vi "Menu Actions.vi"(0 "queue in":refnum<queue>, 1 "LBCB Number":T1, 2 "menu reference":refnum<k9>, 3 "error in":errorcluster, 4 "ItemTag":string) -> (5 "queue out":refnum<queue>, 6 "error out":errorcluster)   [LabVIEW 2009]
uses:
  Data Access Objects/Metadata/LBCB Number.ctl
  Control Loop/Parameters Changes.ctl
  Control Loop/Parameter Change States.ctl
  App Status Actions.ctl
  Launcher/Launcher Actions.ctl
  Launcher/NoPanelAppTypes.ctl
  Data Access Objects/Metadata/Persistant DAO Actions.ctl
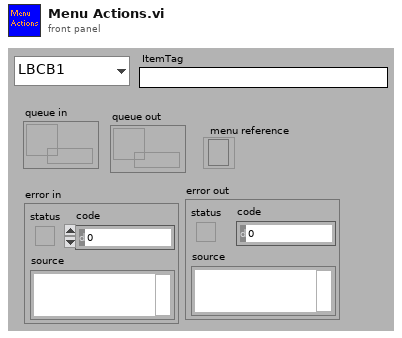
[diagram p1: front panel]
types:
  T1 = typedef "LBCB Number.ctl" = enum16{"LBCB1", "LBCB2"}
  T2 = typedef "Parameters Changes.ctl" = cluster{"Change State":T3, "LBCB Number":T1}
  T3 = typedef "Parameter Change States.ctl" = enum16{"Mixed Mode", "Control Loop", "Limits", "Application", "Stiffness Jacobian", "Start DAQ", "Auto-Balancing", "Set Command", "Enable Control", "Disable Control", "Stop Application"}
  T4 = typedef "App Status Actions.ctl" = enum16{"Init", "Get Status", "Running", "Control", "Autobalanced", "Data Acquisition", "Set App State", "DAQ Started", "Set LBCB State", "Set All", "Set Cont Logging", "Set Step Logging", "Set MM Logging", "Set Volt Logging", "Set Cart Type", "Set DAQ Link", "Set NTCP Link"}
  T5 = typedef "Launcher Actions.ctl" = enum16{"Launch", "Stop All", "Stop", "Kill", "Running?", "Init"}
  T6 = typedef "NoPanelAppTypes.ctl" = enum16{"NTCP Socket", "Data Archiving", "DAQ Link", "Control Loops", "Autobalance Monitor", "Mixed Mode Monitor", "Cmd Disp Diffs"}
  T7 = typedef "Persistant DAO Actions.ctl" = enum16{"Init", "Get", "Set", "Load", "Save"}
  T8 = typedef "LBCB Location.ctl" = enum16{"Crane Bay Two LBCB", "Crane Bay One LBCB", "5th Scale Two LBCB", "5th Scale One LBCB", "Portable LBCB"}
  T9 = typedef "Stiffness Matrix.ctl" = dbl[][]
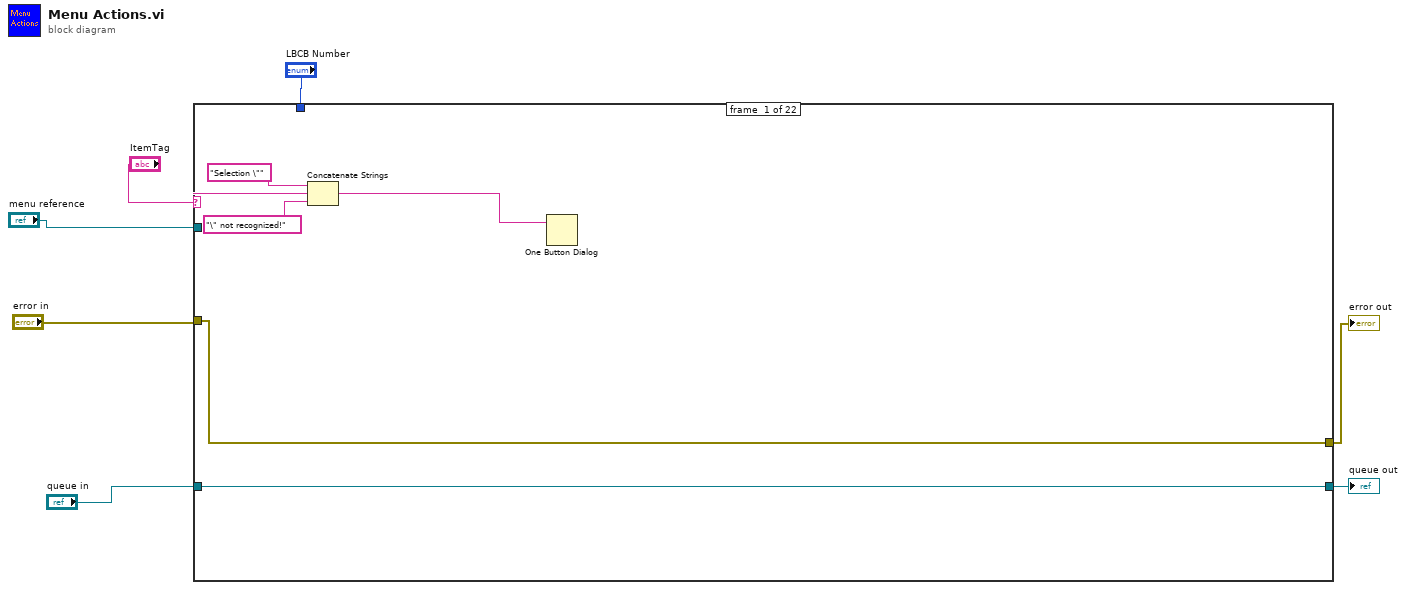
[diagram p0: block diagram]
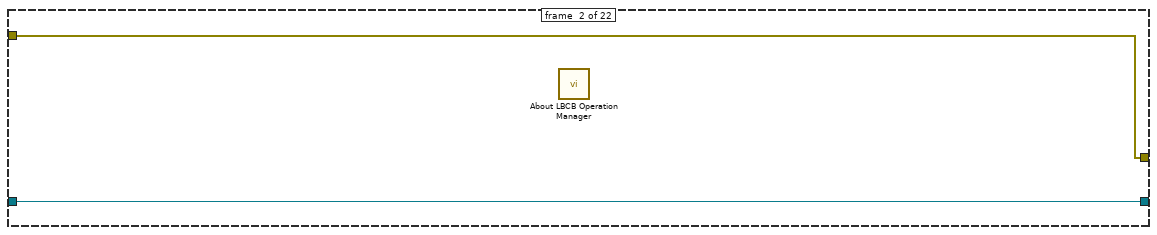
[diagram p2: hidden frame]
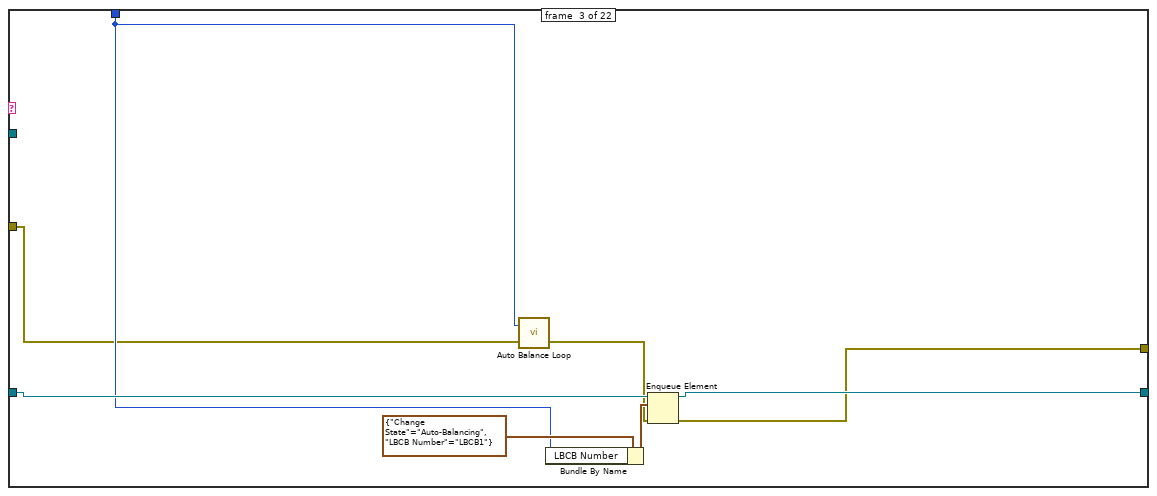
[diagram p3: hidden frame]
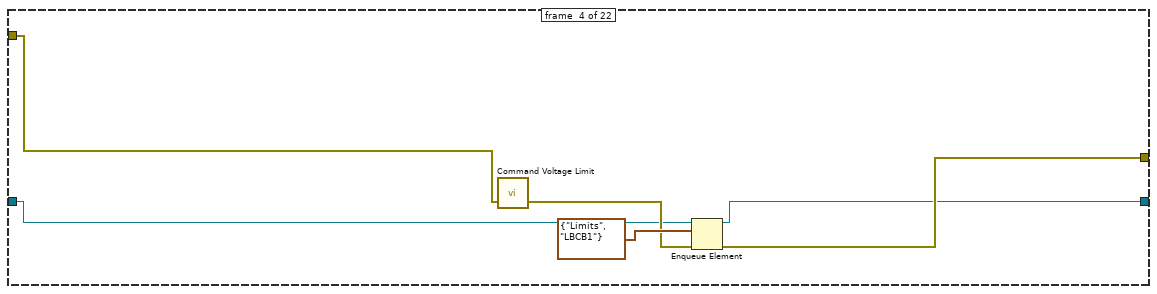
[diagram p4: hidden frame]
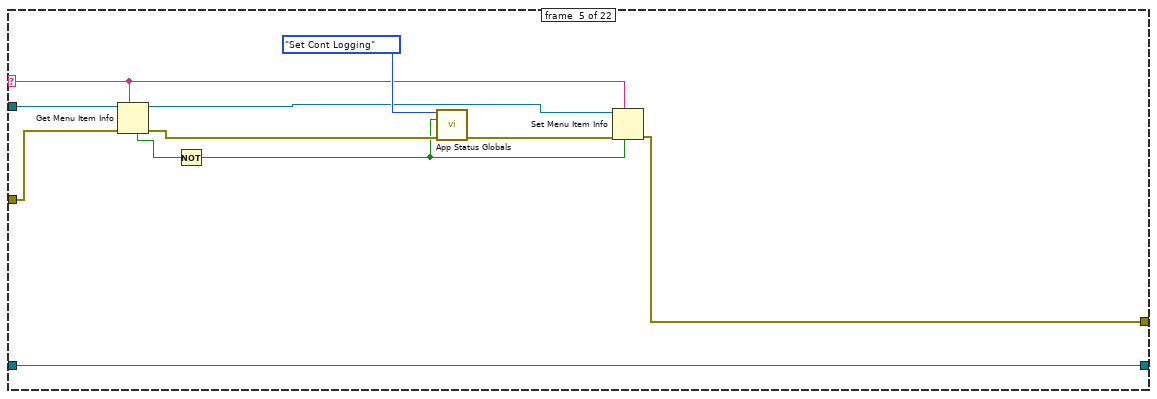
[diagram p5: hidden frame]
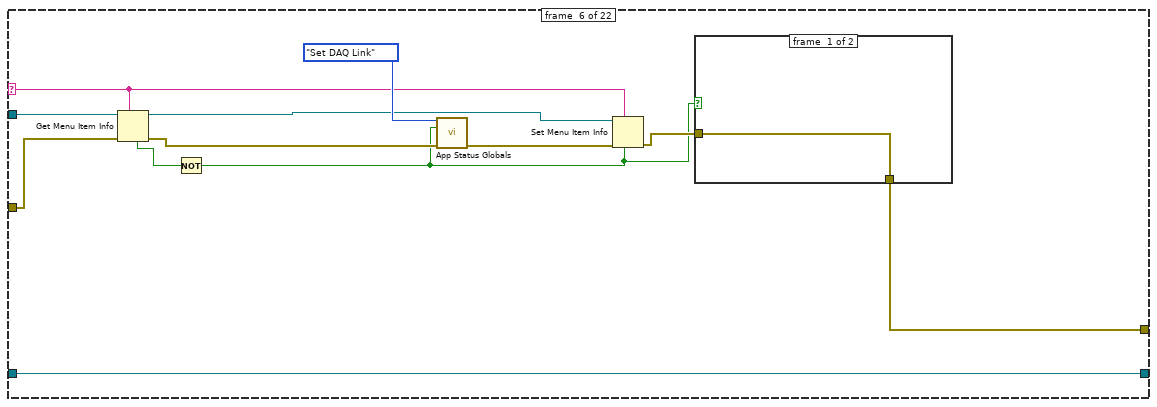
[diagram p6: hidden frame]
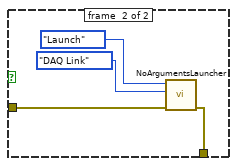
[diagram p7: hidden frame]
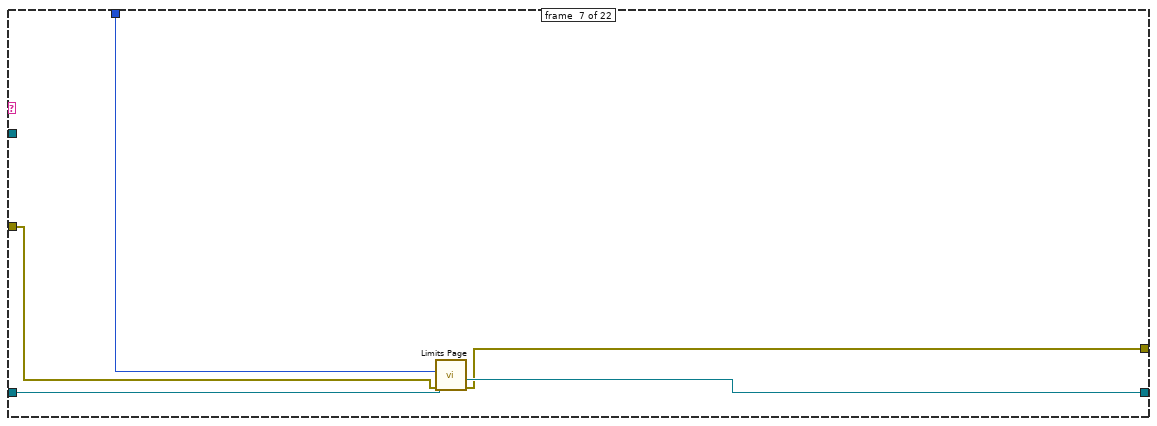
[diagram p8: hidden frame]
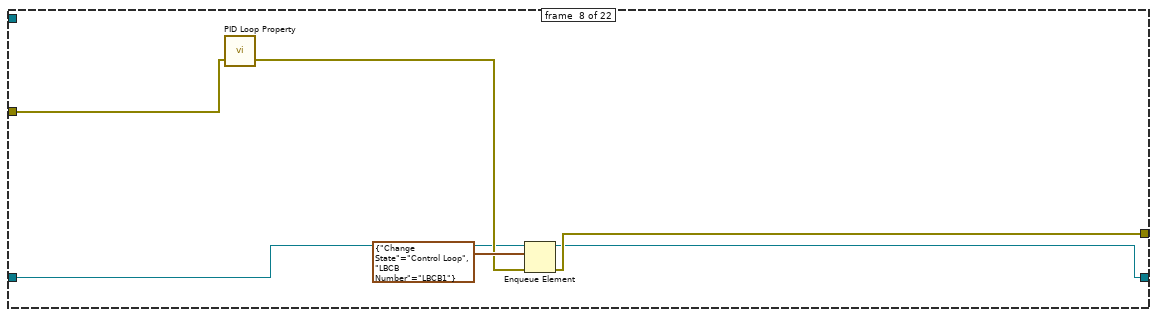
[diagram p9: hidden frame]
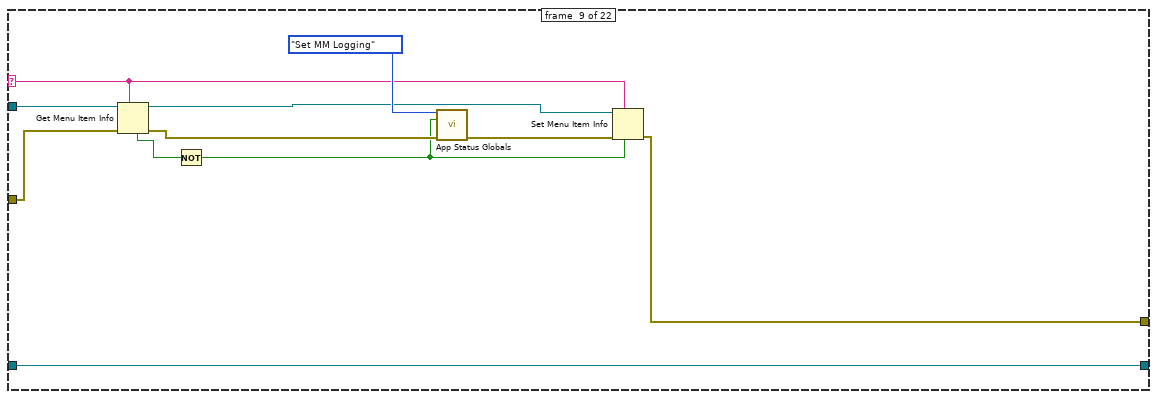
[diagram p10: hidden frame]
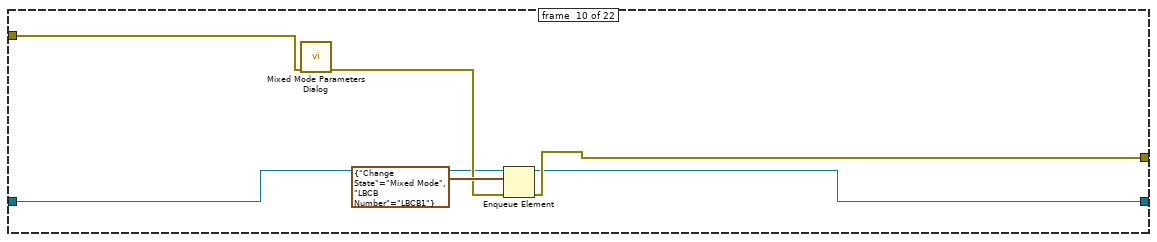
[diagram p11: hidden frame]
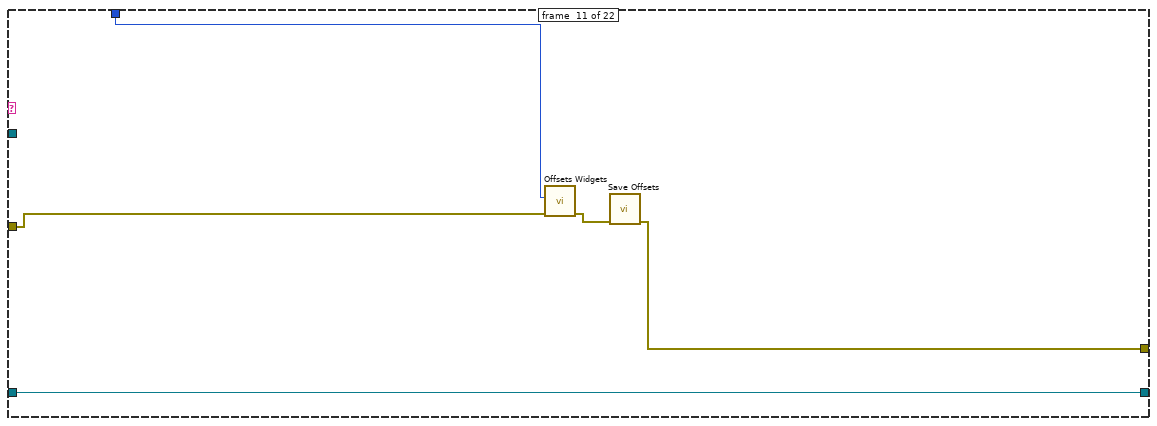
[diagram p12: hidden frame]
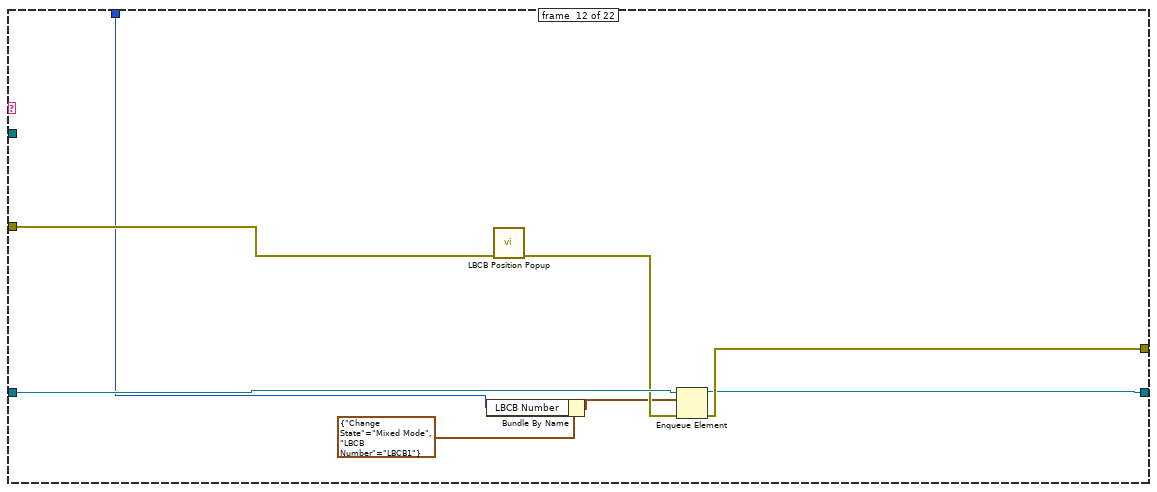
[diagram p13: hidden frame]
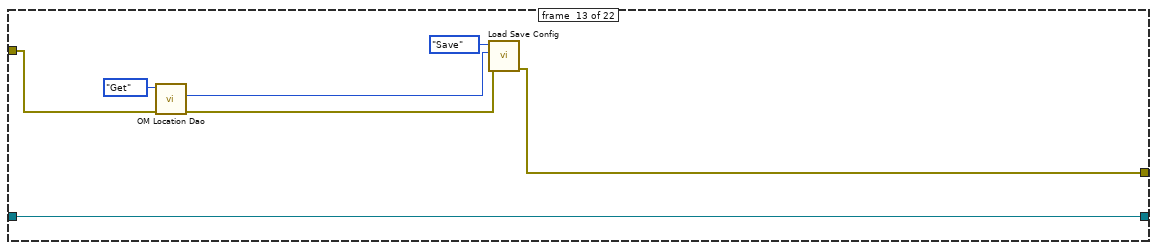
[diagram p14: hidden frame]
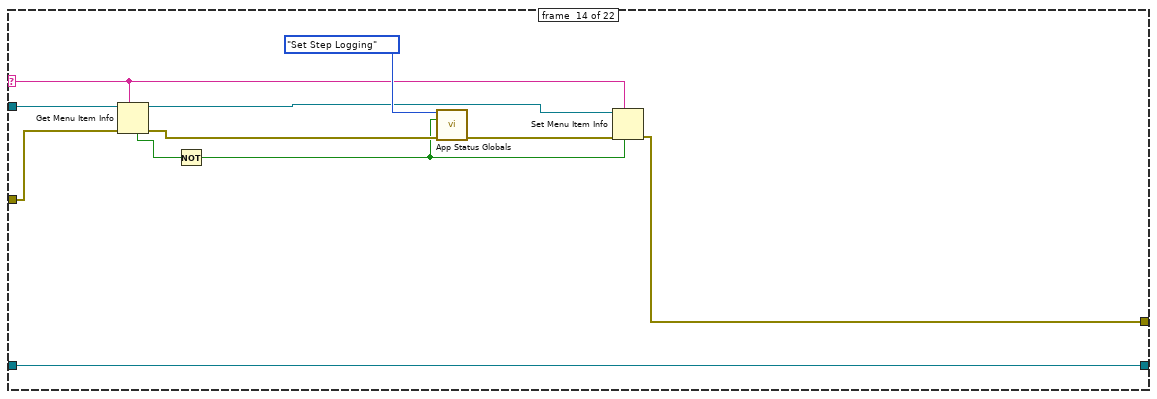
[diagram p15: hidden frame]
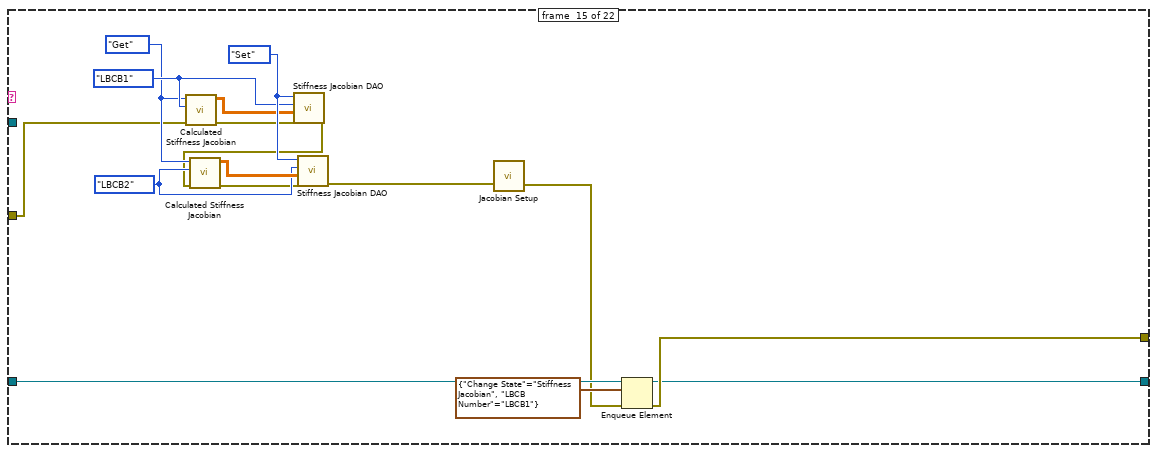
[diagram p16: hidden frame]
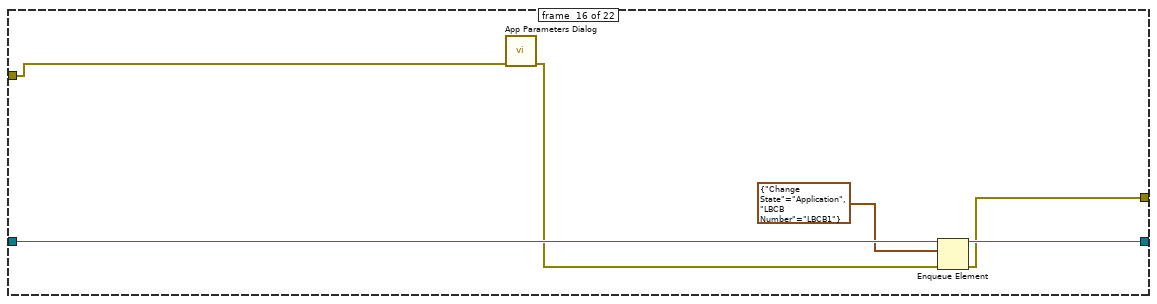
[diagram p17: hidden frame]
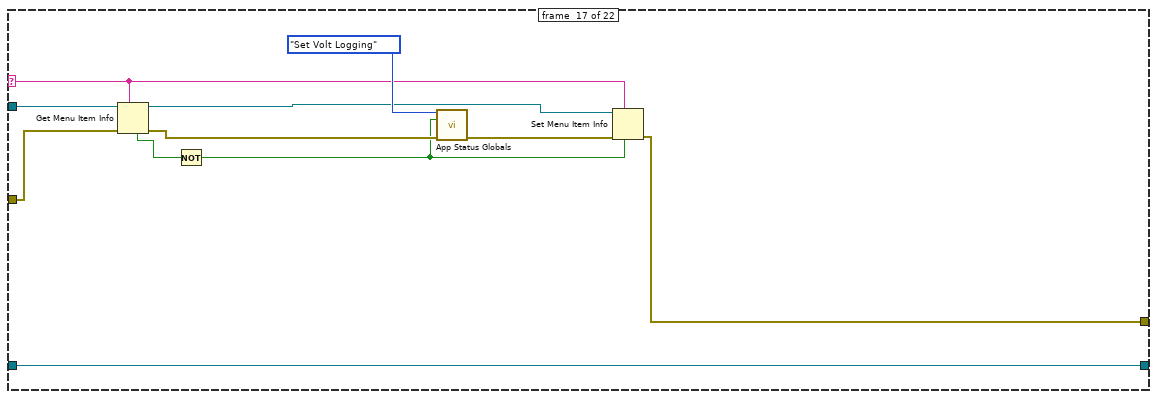
[diagram p18: hidden frame]
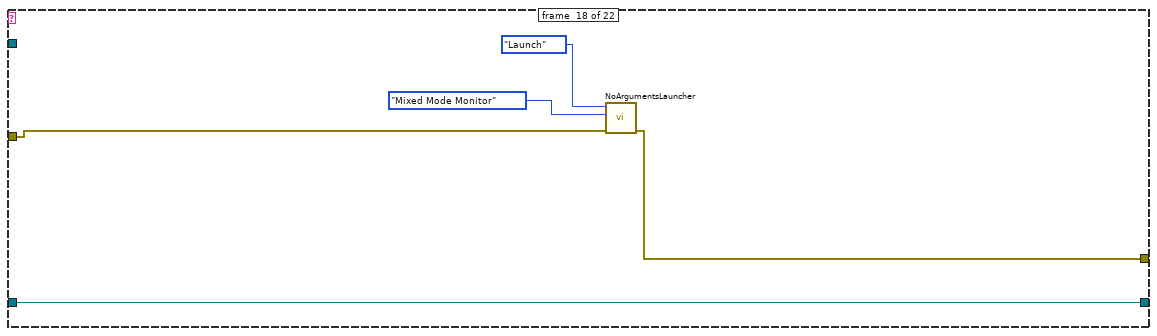
[diagram p19: hidden frame]
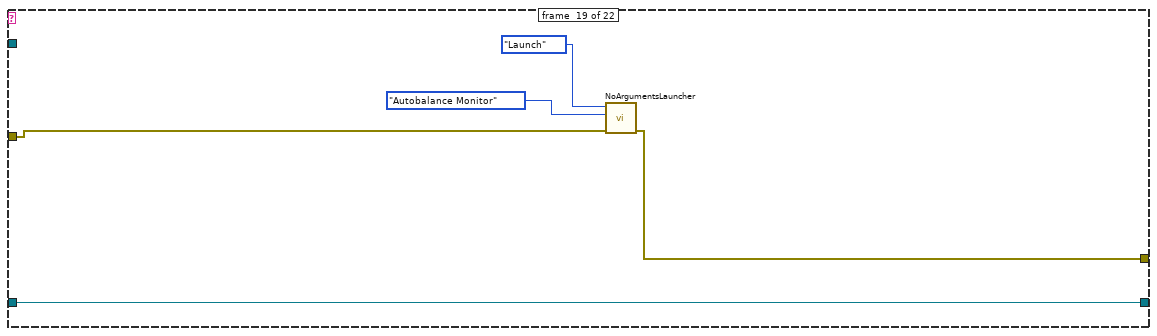
[diagram p20: hidden frame]
diagram:
  n1 = case shown="\"Limits\"" "ItemTag" {
    selector: "ItemTag" -> [w12 _ _ _ w31 w44 _ _ w70 _ _ _ _ w107 _ _ w140 _ _ _ _ _]
    tunnel: [w9 w14 w16 w26 w35 w42 w58 w65 w74 w82 w87 w94 w105 w111 w119 w133 w144 w151 w156 w161 w166 w171] -> w4
    tunnel: "error in" -> [w9 w14 w18 w29 w34 w47 w62 w68 w73 w85 w90 w96 w100 w110 w117 w138 w143 w152 w157 w162 w167 w172]
    tunnel: "queue in" -> [w8 w15 w23 w25 w37 w49 w60 w64 w76 w81 w86 w97 w103 w113 w122 w136 w146 w150 w155 w160 w165 w170]
    tunnel: [w8 w15 w20 w24 w37 w49 w59 w63 w76 w80 w86 w93 w103 w113 w118 w137 w146 w150 w155 w160 w165 w170] -> w6
    tunnel: "LBCB Number" -> [_ _ w19 _ _ _ w61 _ _ _ w89 w91 _ _ _ _ _ _ _ _ _ _]
    tunnel: "menu reference" -> [_ _ _ _ w40 w52 _ _ w79 _ _ _ _ w116 _ _ w149 _ _ _ _ _]
    frame #0 {
      n2 = Concatenate Strings("Selection \"", w12, "\" not recognized!" ("string")) -> (w10:string)
      n3 = One Button Dialog(message=w10) -> ()  [unwired: 2 out]
    }
    frame #1 {
      n4 = call "About LBCB Operation Manager.vi"() -> ()  [unwired: 1 out]
    }
    frame #2 {
      n5 = call "Auto Balance Loop.vi"("error in (no error)"=w18, "LBCB Number"=w19) -> ("error out"=w17:errorcluster)  [unwired: 1 out]
      n6 = Bundle By Name(cluster=T2 {"Change State"=enum."Auto-Balancing", "LBCB Number"=enum."LBCB1"} ("element"), "LBCB Number"=w19) -> (w21:T2)
      n7 = Enqueue Element(queue=w23, element=w21, error in (no error)=w17) -> (queue out=w20:refnum<queue>, error out=w16:errorcluster)  [unwired: 2 out]
    }
    frame #3 {
      n8 = call "Command Voltage Limit.vi"("error in (no error)"=w29) -> ("error out"=w27:errorcluster)  [unwired: 1 in, 1 out]
      n9 = Enqueue Element(queue=w25, element=T2 {"Change State"=enum."Limits", "LBCB Number"=enum."LBCB1"}, error in (no error)=w27) -> (queue out=w24:refnum<queue>, error out=w26:errorcluster)  [unwired: 2 out]
    }
    frame #4 {
      n10 = Get Menu Item Info(7:w31, 8:w34, 11:w40) -> (0:w33:errorcluster, 3:w32:refnum<k9>, 4:w38:bool)  [unwired: 4 out]
      n11 = Not(x=w38) -> (.not. x?=w30:bool)
      n12 = call "App Status Globals.vi"("App Status Actions"=App_Status_Actions."Set Cont Logging", "Status\nSetting"=w30, "error in (no error)"=w33) -> ("error out"=w36:errorcluster)  [unwired: 3 in, 9 out]
      n13 = Set Menu Item Info(6:w30, 7:w31, 8:w36, 11:w32) -> (0:w35:errorcluster)  [unwired: 4 out]
    }
    frame #5 {
      n14 = Get Menu Item Info(7:w44, 8:w47, 11:w52) -> (0:w46:errorcluster, 3:w45:refnum<k9>, 4:w50:bool)  [unwired: 4 out]
      n15 = Not(x=w50) -> (.not. x?=w41:bool)
      n16 = call "App Status Globals.vi"("App Status Actions"=App_Status_Actions."Set DAQ Link", "Status\nSetting"=w41, "error in (no error)"=w46) -> ("error out"=w48:errorcluster)  [unwired: 3 in, 9 out]
      n17 = Set Menu Item Info(6:w41, 7:w44, 8:w48, 11:w45) -> (0:w43:errorcluster)  [unwired: 4 out]
      n18 = case shown="False" w41 {
        tunnel: w43 -> [w53 w55]
        tunnel: [w53 w54] -> w42
        frame #0 {
        }
        frame #1 {
          n19 = call "NoArgumentsLauncher.vi"("error in (no error)"=w55, "Application"=NoPanelAppTypes."DAQ Link", "Application Launcher Actions"=Launcher_Actions."Launch") -> ("error out"=w54:errorcluster)  [unwired: 8 out]
        }
      }
    }
    frame #6 {
      n20 = call "Limits Page.vi"("error in (no error)"=w62, "queue in"=w60, "LBCB Number"=w61) -> ("error out"=w58:errorcluster, "queue out"=w59:refnum<queue>)  [unwired: 7 in]
    }
    frame #7 {
      n21 = call "PID Loop Property.vi"("error in (no error)"=w68) -> ("error out"=w66:errorcluster)  [unwired: 1 in, 1 out]
      n22 = Enqueue Element(queue=w64, element=T2 {"Change State"=enum."Control Loop", "LBCB Number"=enum."LBCB1"}, error in (no error)=w66) -> (queue out=w63:refnum<queue>, error out=w65:errorcluster)  [unwired: 2 out]
    }
    frame #8 {
      n23 = Get Menu Item Info(7:w70, 8:w73, 11:w79) -> (0:w72:errorcluster, 3:w71:refnum<k9>, 4:w77:bool)  [unwired: 4 out]
      n24 = Not(x=w77) -> (.not. x?=w69:bool)
      n25 = call "App Status Globals.vi"("App Status Actions"=App_Status_Actions."Set MM Logging", "Status\nSetting"=w69, "error in (no error)"=w72) -> ("error out"=w75:errorcluster)  [unwired: 3 in, 9 out]
      n26 = Set Menu Item Info(6:w69, 7:w70, 8:w75, 11:w71) -> (0:w74:errorcluster)  [unwired: 4 out]
    }
    frame #9 {
      n27 = call "Mixed Mode Parameters Dialog.vi"("error in (no error)"=w85) -> ("error out"=w83:errorcluster)  [unwired: 1 in, 9 out]
      n28 = Enqueue Element(queue=w81, element=T2 {"Change State"=enum."Mixed Mode", "LBCB Number"=enum."LBCB1"}, error in (no error)=w83) -> (queue out=w80:refnum<queue>, error out=w82:errorcluster)  [unwired: 2 out]
    }
    frame #10 {
      n29 = call "Offsets Widgets.vi"("error in (no error)"=w90, "LBCB Selected"=w89) -> ("error out"=w88:errorcluster)  [unwired: 9 out]
      n30 = call "Save Offsets.vi"("error in (no error)"=w88) -> ("error out"=w87:errorcluster)  [unwired: 10 out]
    }
    frame #11 {
      n31 = Bundle By Name(cluster=T2 {"Change State"=enum."Mixed Mode", "LBCB Number"=enum."LBCB1"} ("element"), "LBCB Number"=w91) -> (w92:T2)
      n32 = call "LBCB Position Popup.vi"("error in (no error)"=w96) -> ("error out"=w95:errorcluster)  [unwired: 1 in, 9 out]
      n33 = Enqueue Element(queue=w97, element=w92, error in (no error)=w95) -> (queue out=w93:refnum<queue>, error out=w94:errorcluster)  [unwired: 2 out]
    }
    frame #12 {
      n34 = call "OM Location Dao.vi"("error in (no error)"=w100, "Actions"=Persistant_DAO_Actions."Get") -> ("error out"=w99:errorcluster, "LBCB  Location Out"=w101:T8)  [unwired: 2 in, 6 out]
      n35 = call "Load Save Config.vi"("error in (no error)"=w99, "OM  Location"=w101, "Actions"=Persistant_DAO_Actions."Save") -> ("error out"=w105:errorcluster)  [unwired: 8 out]
    }
    frame #13 {
      n36 = Get Menu Item Info(7:w107, 8:w110, 11:w116) -> (0:w109:errorcluster, 3:w108:refnum<k9>, 4:w114:bool)  [unwired: 4 out]
      n37 = Not(x=w114) -> (.not. x?=w106:bool)
      n38 = call "App Status Globals.vi"("App Status Actions"=App_Status_Actions."Set Step Logging", "Status\nSetting"=w106, "error in (no error)"=w109) -> ("error out"=w112:errorcluster)  [unwired: 3 in, 9 out]
      n39 = Set Menu Item Info(6:w106, 7:w107, 8:w112, 11:w108) -> (0:w111:errorcluster)  [unwired: 4 out]
    }
    frame #14 {
      w131 = Persistant_DAO_Actions."Set" ("Actions")
      w128 = LBCB_Number."LBCB1" ("LBCB Number")
      w129 = LBCB_Number."LBCB2" ("LBCB Number")
      w127 = Persistant_DAO_Actions."Get" ("Actions")
      n40 = call "Calculated Stiffness Jacobian.vi"("error in (no error)"=w117, "LBCB Number"=w128, "Actions"=w127) -> ("error out"=w126:errorcluster, "Stiffness Jacobian Out"=w130:T9)  [unwired: 1 in, 6 out]
      n41 = call "Stiffness Jacobian DAO.vi"("error in (no error)"=w126, "Stiffness Jacobian In"=w130, "LBCB Number"=w128, "Actions"=w131) -> ("error out"=w124:errorcluster)  [unwired: 1 in, 6 out]
      n42 = call "Calculated Stiffness Jacobian.vi"("error in (no error)"=w124, "LBCB Number"=w129, "Actions"=w127) -> ("error out"=w125:errorcluster, "Stiffness Jacobian Out"=w132:T9)  [unwired: 1 in, 6 out]
      n43 = call "Stiffness Jacobian DAO.vi"("error in (no error)"=w125, "Stiffness Jacobian In"=w132, "LBCB Number"=w129, "Actions"=w131) -> ("error out"=w123:errorcluster)  [unwired: 1 in, 6 out]
      n44 = call "Jacobian Setup.vi"("error in (no error)"=w123) -> ("error out"=w120:errorcluster)  [unwired: 1 in, 1 out]
      n45 = Enqueue Element(queue=w122, element=T2 {"Change State"=enum."Stiffness Jacobian", "LBCB Number"=enum."LBCB1"}, error in (no error)=w120) -> (queue out=w118:refnum<queue>, error out=w119:errorcluster)  [unwired: 2 out]
    }
    frame #15 {
      n46 = call "App Parameters Dialog.vi"("error in (no error)"=w138) -> ("error out"=w134:errorcluster)  [unwired: 10 out]
      n47 = Enqueue Element(queue=w136, element=T2 {"Change State"=enum."Application", "LBCB Number"=enum."LBCB1"}, error in (no error)=w134) -> (queue out=w137:refnum<queue>, error out=w133:errorcluster)  [unwired: 2 out]
    }
    frame #16 {
      n48 = Get Menu Item Info(7:w140, 8:w143, 11:w149) -> (0:w142:errorcluster, 3:w141:refnum<k9>, 4:w147:bool)  [unwired: 4 out]
      n49 = Not(x=w147) -> (.not. x?=w139:bool)
      n50 = call "App Status Globals.vi"("App Status Actions"=App_Status_Actions."Set Volt Logging", "Status\nSetting"=w139, "error in (no error)"=w142) -> ("error out"=w145:errorcluster)  [unwired: 3 in, 9 out]
      n51 = Set Menu Item Info(6:w139, 7:w140, 8:w145, 11:w141) -> (0:w144:errorcluster)  [unwired: 4 out]
    }
    frame #17 {
      n52 = call "NoArgumentsLauncher.vi"("error in (no error)"=w152, "Application"=NoPanelAppTypes."Mixed Mode Monitor", "Application Launcher Actions"=Launcher_Actions."Launch") -> ("error out"=w151:errorcluster)  [unwired: 8 out]
    }
    frame #18 {
      n53 = call "NoArgumentsLauncher.vi"("error in (no error)"=w157, "Application"=NoPanelAppTypes."Autobalance Monitor", "Application Launcher Actions"=Launcher_Actions."Launch") -> ("error out"=w156:errorcluster)  [unwired: 8 out]
    }
    frame #19 {
      n54 = call "NoArgumentsLauncher.vi"("error in (no error)"=w162, "Application"=NoPanelAppTypes."Cmd Disp Diffs", "Application Launcher Actions"=Launcher_Actions."Launch") -> ("error out"=w161:errorcluster)  [unwired: 8 out]
    }
    frame #20 {
      n55 = call "NoArgumentsLauncher.vi"("error in (no error)"=w167, "Application"=NoPanelAppTypes."Cmd Disp Diffs", "Application Launcher Actions"=Launcher_Actions."Launch") -> ("error out"=w166:errorcluster)  [unwired: 8 out]
    }
    frame #21 {
      n56 = call "NoArgumentsLauncher.vi"("error in (no error)"=w172, "Application"=NoPanelAppTypes."NTCP Socket", "Application Launcher Actions"=Launcher_Actions."Launch") -> ("error out"=w171:errorcluster)  [unwired: 8 out]
    }
  }
  "queue out" <- w6
  "error out" <- w4
